vi "Homography UnitX Matrix C.vi"(1 "input cluster":T1) -> (0 "C":T2)   [LabVIEW 2015]
uses:
  <vilib>/Analysis/Matrix/Datatypes/RealMatrix.ctl
  <vilib>/Analysis/baseanly.llb/Real A x B.vi
  <vilib>/Analysis/Matrix/Numeric/Conversions/Matrix To Array - RM.vi
  <vilib>/Analysis/baseanly.llb/Real Inverse Matrix.vi
  <vilib>/Analysis/Matrix/Numeric/Conversions/Array To Matrix - RA2.vi
  <vilib>/Analysis/Matrix/NI_Matrix.lvlib
  <vilib>/Analysis/NI_AALBase.lvlib
panel:
  out "inv(A) 2":T2
  out "inv(A)":T2
  out "Image Factors 2":T2
  out "Image Inverse Matrix 2":T2
  out "Column 2":T2
  out "temp 2":T2
  out "Input 2":T2
  out "B":T2
  out "Image Factors":T2
  out "Image Inverse Matrix":T2
  out "Column":T2
  out "temp":T2
  out "Input":T2
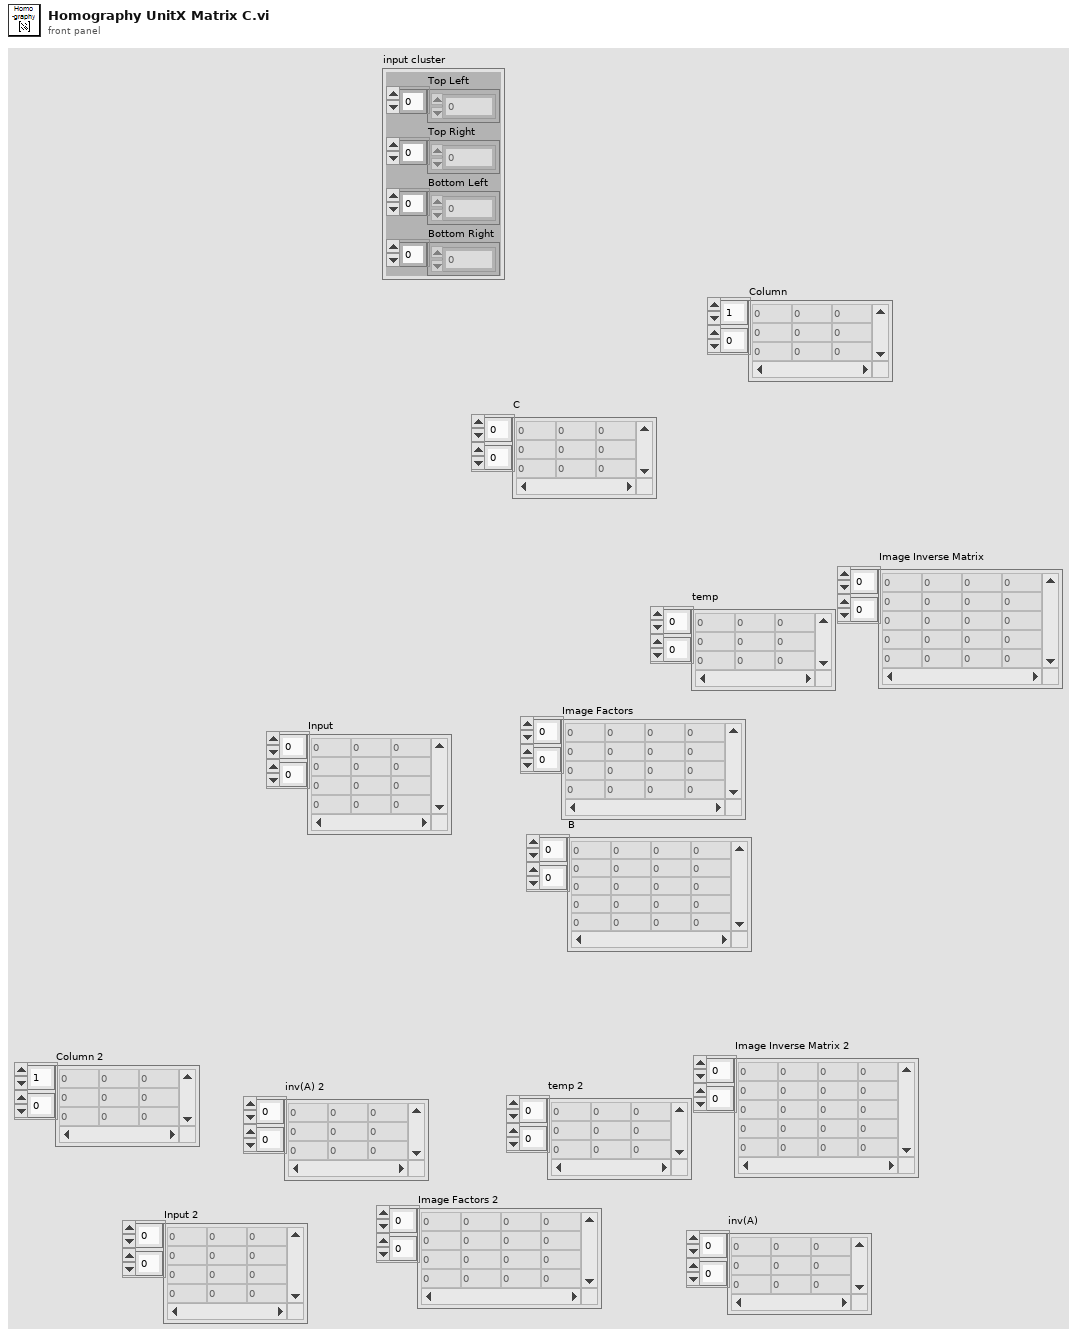
[diagram p1: front panel]
types:
  T1 = cluster{"Top Left":dbl[], "Top Right":dbl[], "Bottom Left":dbl[], "Bottom Right":dbl[]}
  T2 = typedef "NI_Matrix.lvlib/RealMatrix.ctl" = dbl[][]
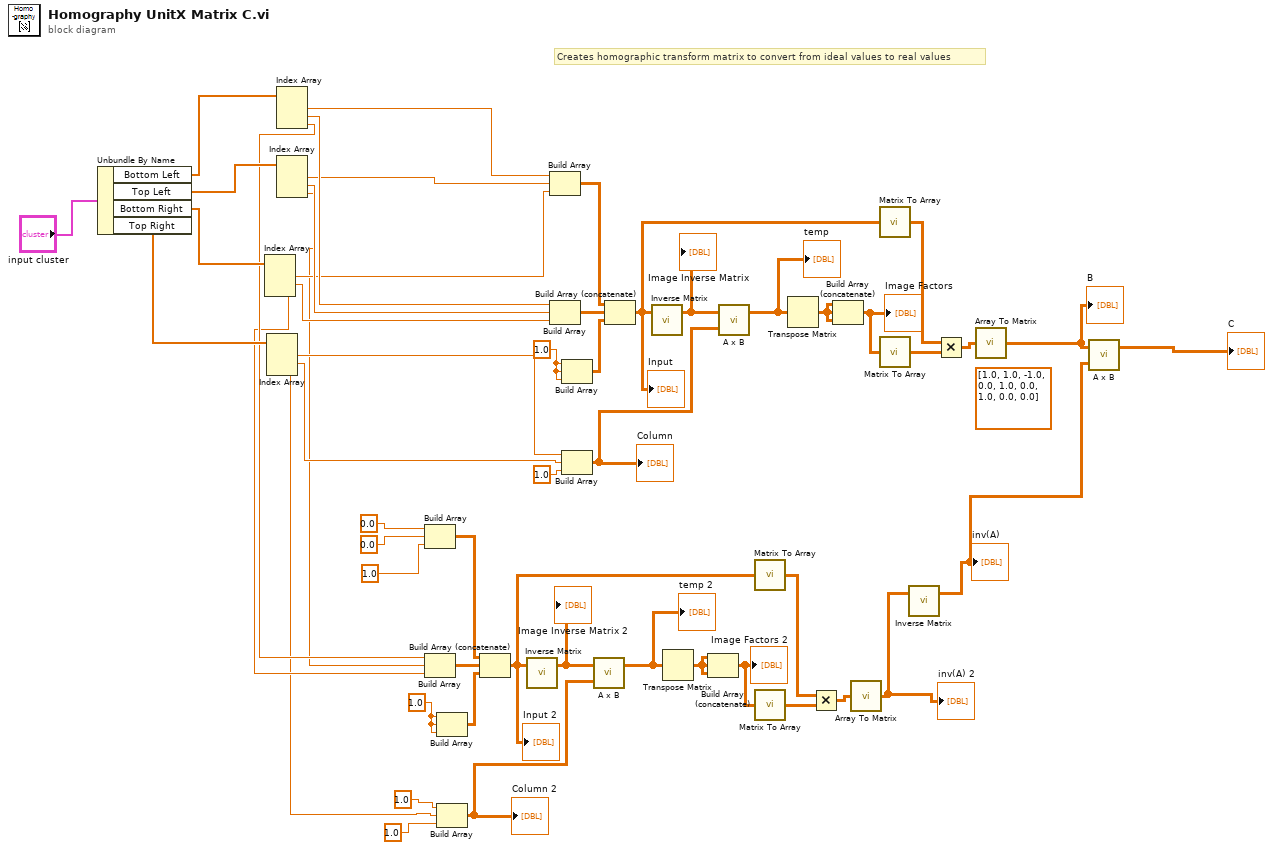
[diagram p0: block diagram]
diagram:
  w25 = 1.0 ("index (row)")
  (unwired) T2 [[1.0, 1.0, -1.0], [0.0, 1.0, 0.0], [1.0, 0.0, 0.0]] ("appended array")
  w53 = 1.0 ("index (row)")
  # "Creates homographic transform matrix to convert from ideal values to real values"
  n1 = Unbundle By Name("input cluster") -> ("Bottom Left"=w37:dbl[], "Top Left"=w34:dbl[], "Bottom Right"=w31:dbl[], "Top Right"=w28:dbl[])
  n2 = Index Array(array=w31) -> (element #1=w30:dbl, element #2=w29:dbl, element #3=w7:dbl)  [unwired: 3 in]
  n3 = Index Array(array=w28) -> (element #1=w27:dbl, element #2=w26:dbl, element #3=w5:dbl)  [unwired: 3 in]
  n4 = Index Array(array=w37) -> (element #1=w36:dbl, element #2=w35:dbl, element #3=w9:dbl)  [unwired: 3 in]
  n5 = Index Array(array=w34) -> (element #1=w33:dbl, element #2=w32:dbl, element #3=w8:dbl)  [unwired: 3 in]
  n6 = Build Array(0.0, 0.0, 1.0) -> (w24:T2)
  n7 = Build Array(w9, w8, w7) -> (w23:T2)
  n8 = Build Array(w25, w25, w25) -> (w22:T2)
  n9 = Build Array(1.0 ("index (row)"), w5, 1.0 ("index (row)")) -> (w21:T2)
  "Column 2" <- w21
  n10 = Build Array (concatenate)(w24, w23, w22) -> (w17:T2)
  "Input 2" <- w17
  n11 = call-poly <vilib>:"Inverse Matrix.vi"("Input Matrix"=w17) -> ("Inverse Matrix"=w18:T2)  [unwired: 1 in, 1 out]
  "Image Inverse Matrix 2" <- w18
  n12 = Build Array(w36, w33, w30) -> (w52:T2)
  n13 = Build Array(w35, w32, w29) -> (w51:T2)
  n14 = Build Array(w53, w53, w53) -> (w50:T2)
  n15 = Build Array(w27, w26, 1.0 ("index (row)")) -> (w48:T2)
  "Column" <- w48
  n16 = call-poly <vilib>:"A x B.vi"("B"=w21, "A"=w18) -> ("A x B"=w20:T2)  [unwired: 1 out]
  "temp 2" <- w20
  n17 = Build Array (concatenate)(w52, w51, w50) -> (w44:T2)
  "Input" <- w44
  n18 = call-poly <vilib>:"Inverse Matrix.vi"("Input Matrix"=w44) -> ("Inverse Matrix"=w45:T2)  [unwired: 1 in, 1 out]
  "Image Inverse Matrix" <- w45
  n19 = Transpose Matrix(1:w20) -> (0:w19:T2)
  n20 = Build Array (concatenate)(w19, w19, w19) -> (w13:T2)
  "Image Factors 2" <- w13
  n21 = call-poly <vilib>:"A x B.vi"("B"=w48, "A"=w45) -> ("A x B"=w47:T2)  [unwired: 1 out]
  "temp" <- w47
  n22 = call-poly <vilib>:"Matrix To Array.vi"("Real Matrix"=w17) -> ("Real 2D Array"=w16:dbl[][])
  n23 = call-poly <vilib>:"Matrix To Array.vi"("Real Matrix"=w13) -> ("Real 2D Array"=w14:dbl[][])
  n24 = Transpose Matrix(1:w47) -> (0:w46:T2)
  n25 = Multiply(x=w16, y=w14) -> (x*y=w15:dbl[][])
  n26 = Build Array (concatenate)(w46, w46, w46) -> (w40:T2)
  "Image Factors" <- w40
  n27 = call-poly <vilib>:"Array To Matrix.vi"("Real 2D Array"=w15) -> ("Real Matrix"=w4:T2)
  "inv(A) 2" <- w4
  n28 = call-poly <vilib>:"Matrix To Array.vi"("Real Matrix"=w44) -> ("Real 2D Array"=w43:dbl[][])
  n29 = call-poly <vilib>:"Matrix To Array.vi"("Real Matrix"=w40) -> ("Real 2D Array"=w41:dbl[][])
  n30 = call-poly <vilib>:"Inverse Matrix.vi"("Input Matrix"=w4) -> ("Inverse Matrix"=w3:T2)  [unwired: 1 in, 1 out]
  "inv(A)" <- w3
  n31 = Multiply(x=w43, y=w41) -> (x*y=w42:dbl[][])
  n32 = call-poly <vilib>:"Array To Matrix.vi"("Real 2D Array"=w42) -> ("Real Matrix"=w39:T2)
  "B" <- w39
  n33 = call-poly <vilib>:"A x B.vi"("B"=w3, "A"=w39) -> ("A x B"=→"C":T2)  [unwired: 1 out]
